vi "ep05_advanced_digital_signal_generator.vi"() -> ()   [LabVIEW 2019]
panel:
  in  "stop":bool
  out "Service Status":bool
  out "Port Status":bool
  out "Information":string="err: Could not open the port \"COM1\"\r\n"
  in  "Baud Rate":T1(ring)=enum."115200"
  in  "Port Id":T2(ring)=enum."COM3" caption="Port Name"
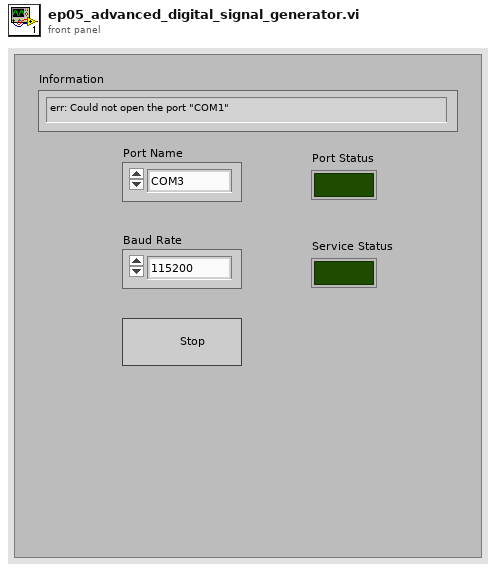
[diagram p1: front panel]
types:
  T1 = enum32{"300", "600", "1200", "2400", "4800", "9600", "14400", "19200", "28800", "38400", "56000", "57600", "115200", "128000", "256000"}
  T2 = enum8{"COM1", "COM2", "COM3", "COM4", "COM5", "COM6", "COM7", "COM8", "COM9", "COM10", "COM11", "COM12", "COM13", "COM14", "COM15", "COM16", "COM17", "COM18", "COM19", "COM20", "COM21", "COM22", "COM23", "COM24", "COM25", "COM26", "COM27", "COM28", "COM29", "COM30", "COM31", "COM32", "COM33", "COM34", "COM35", "COM36", "COM37", "COM38", "COM39", "COM40", "COM41", "COM42", "COM43", "COM44", "COM45", "COM46", "COM47", "COM48"}
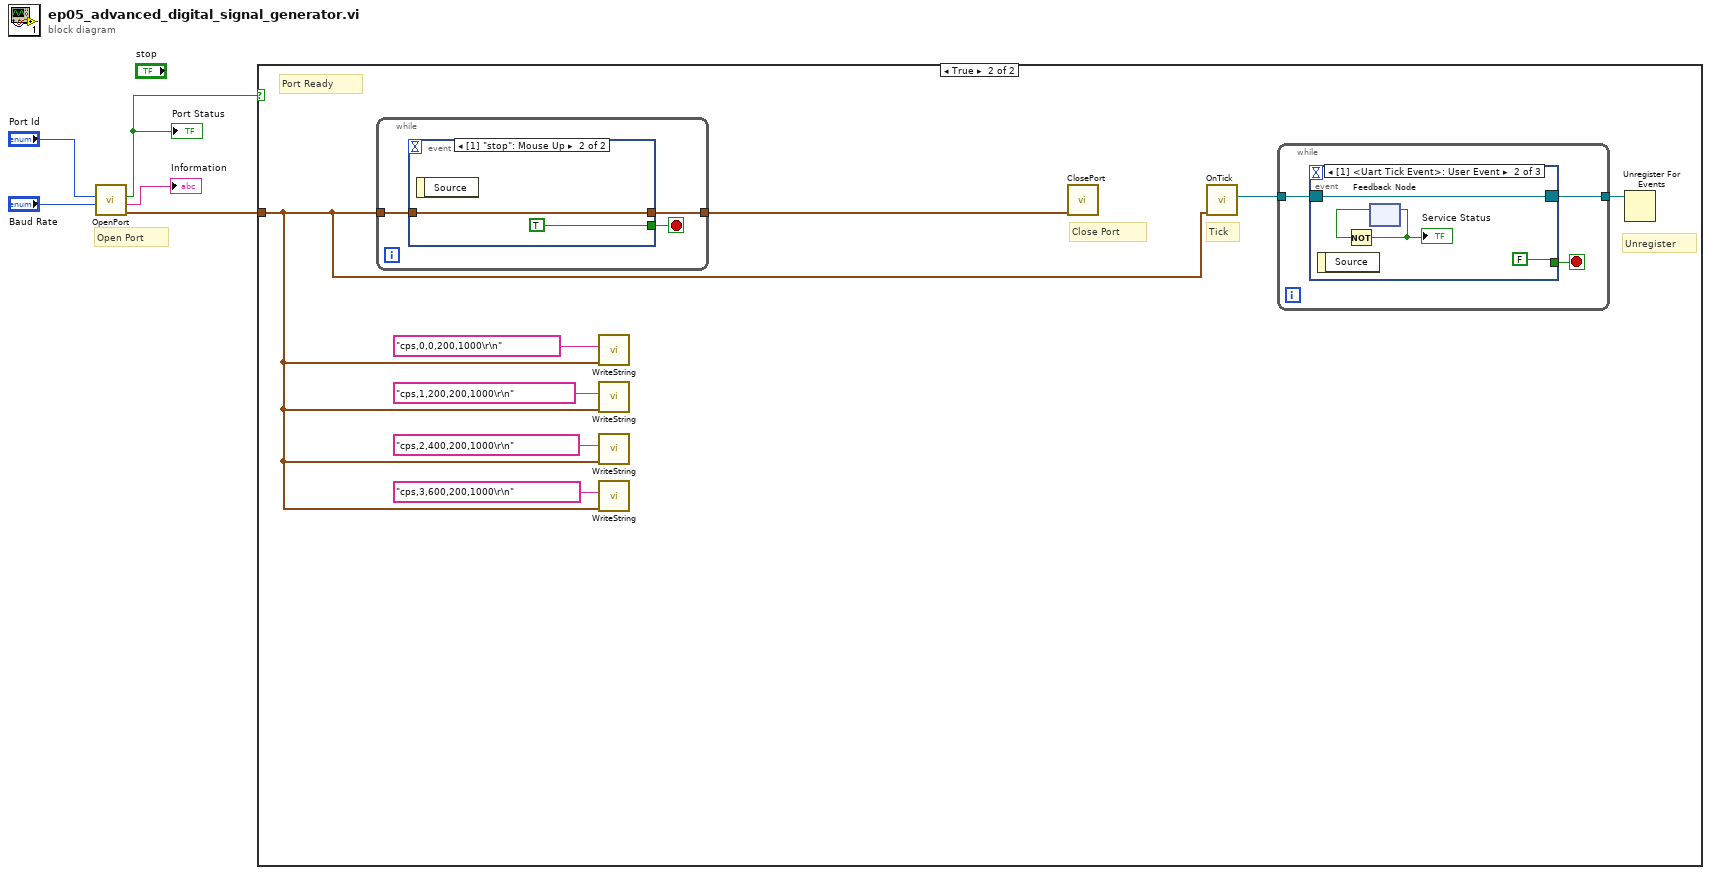
[diagram p0: block diagram]
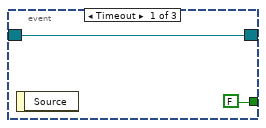
[diagram p3: hidden frame]
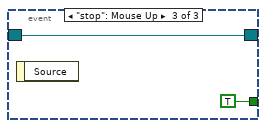
[diagram p4: hidden frame]
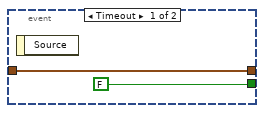
[diagram p5: hidden frame]
diagram:
  # "Open Port"
  n1 = call "OpenPort.vi"("Baud Rate Input"="Baud Rate", "Port Id Input"="Port Id") -> ("Uart Output"=w1:cluster{u64}, "Information"=→"Information":string, "Port Status"=w2:bool)  [unwired: 6 in, 1 out]
  "Port Status" <- w2
  n2 = case shown="True" w2 {
    tunnel: w1 -> [_ w6]
    frame False {
      # "Do nothing"
    }
    frame True {
      # "Unregister"
      # "Close Port"
      # "Tick"
      # "Port Ready"
      n3 = while {
        tunnel: w6 -> [w26]
        tunnel: [w25] -> w11
        stop <- w27 stop-if-true
        n4 = event shown="[1] \"stop\": Mouse Up" {
          selector: _ -> [_ _]
          dyn-events: _ -> [_ _]
          timeout: _ -> [_ _]
          tunnel: [FALSE TRUE] -> w27
          tunnel: w26 -> [w28 w30]
          tunnel: [w28 w30] -> w25
          event Timeout {
            n5 = event-data() -> ()  [unwired: 1 in, 1 out]
          }
          event "stop": Mouse Up {
            n6 = event-data() -> ()  [unwired: 1 in, 1 out]
          }
        }
      }
      n7 = call "WriteString.vi"("Uart Input"=w6, "String Data"="cps,0,0,200,1000\r\n") -> ()  [unwired: 7 in, 3 out]
      n8 = call "WriteString.vi"("Uart Input"=w6, "String Data"="cps,1,200,200,1000\r\n") -> ()  [unwired: 7 in, 3 out]
      n9 = call "WriteString.vi"("Uart Input"=w6, "String Data"="cps,2,400,200,1000\r\n") -> ()  [unwired: 7 in, 3 out]
      n10 = call "WriteString.vi"("Uart Input"=w6, "String Data"="cps,3,600,200,1000\r\n") -> ()  [unwired: 7 in, 3 out]
      n11 = call "ClosePort.vi"("Uart Input"=w11) -> ()  [unwired: 9 in, 2 out]
      n12 = call "OnTick.vi"("Uart Input"=w6) -> ("On Tick Event"=w13:refnum<event-registration>)  [unwired: 8 in, 2 out]
      n13 = while {
        tunnel: w13 -> [w15]
        tunnel: [w14] -> w12
        stop <- w16 stop-if-true
        n14 = event shown="[1] <Uart Tick Event>: User Event" {
          selector: w15 -> [w17 w19 w23]
          dyn-events: [w17 w19 w23] -> w14
          timeout: _ -> [_ _ _]
          tunnel: [FALSE FALSE TRUE] -> w16
          event Timeout {
            n15 = event-data() -> ()  [unwired: 1 in, 1 out]
          }
          event User Event {
            n16 = event-data() -> ()  [unwired: 1 in, 1 out]
            n17 = feedback #1() -> (w21:bool)  [unwired: 1 in]
            n18 = Not(x=w21) -> (.not. x?=w20:bool)
            "Service Status" <- w20
            n19 = feedback-in #1(w20) -> ()
          }
          event "stop": Mouse Up {
            n20 = event-data() -> ()  [unwired: 1 in, 1 out]
          }
        }
      }
      n21 = Unregister For Events(event registration refnum=w12) -> ()  [unwired: 1 in, 1 out]
    }
  }
